vi "windows_heater_safety.vi"(1 "Stop!":refnum<vi>, 2 "Minimum Flow Rate Refnum":refnum<vi>, 3 "Liquid Flow Rate Refnum":refnum<vi>, 4 "Vapor Flow Rate Refnum":refnum<vi>, 5 "Safety Trigger Refnum":refnum<vi>, 6 "Switch Refnum":refnum<vi>) -> ()   [LabVIEW 2016]
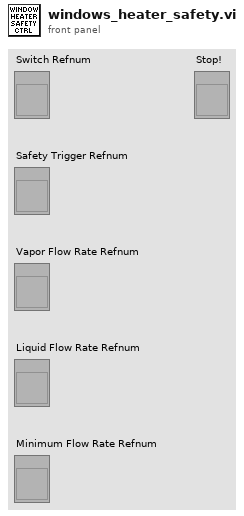
[diagram p1: front panel]
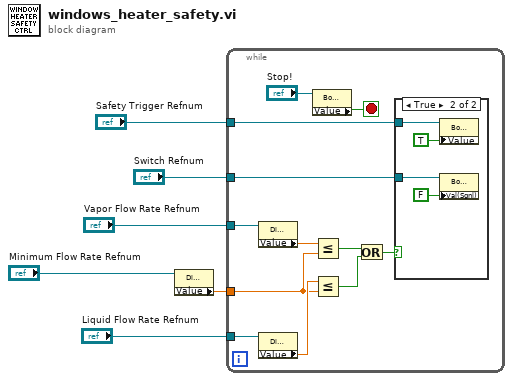
[diagram p0: block diagram]
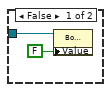
[diagram p2: hidden frame]
diagram:
  n1 = property class="DigNum (strict)"(reference="Minimum Flow Rate Refnum") -> ("Value"=w3:dbl)  [unwired: 1 in, 2 out]
  n2 = while {
    tunnel: "Vapor Flow Rate Refnum" -> [w18]
    tunnel: "Liquid Flow Rate Refnum" -> [w17]
    tunnel: w3 -> [w14]
    tunnel: "Switch Refnum" -> [w8]
    tunnel: "Safety Trigger Refnum" -> [w7]
    stop <- w10 stop-if-true
    n3 = property class="DigNum (strict)"(reference=w18) -> ("Value"=w16:dbl)  [unwired: 1 in, 2 out]
    n4 = property class="DigNum (strict)"(reference=w17) -> ("Value"=w15:dbl)  [unwired: 1 in, 2 out]
    n5 = property class="Bool (strict)"(reference="Stop!") -> ("Value"=w10:bool)  [unwired: 1 in, 2 out]
    n6 = Less Or Equal?(x=w16, y=w14) -> (x <= y?=w13:bool)
    n7 = Less Or Equal?(x=w15, y=w14) -> (x <= y?=w12:bool)
    n8 = Or(x=w13, y=w12) -> (x .or. y?=w9:bool)
    n9 = case shown="True" w9 {
      tunnel: w8 -> [_ w23]
      tunnel: w7 -> [w19 w21]
      frame False {
        n10 = property class="Bool (strict)"(reference=w19, "Value"=FALSE) -> ()  [unwired: 1 in, 2 out]
      }
      frame True {
        n11 = property class="Bool (strict)"(reference=w21, "Value"=TRUE) -> ()  [unwired: 1 in, 2 out]
        n12 = property class="Bool (strict)"(reference=w23, "Val(Sgnl)"=FALSE ("Value")) -> ()  [unwired: 1 in, 2 out]
      }
    }
  }
